vi "Push_OnlyPump.vi"(6 "Control":enum16{"First", "Second"}(ring), 10 "Port 1 in":T1={"Давление заданное"=0.3, "Давление MAX заданное"=100.0, "Давление в насосе"=0.0, "Давление в системе"=99.99, "Расход заданый"=0.0, "Расход текущий"=0.0, "Объём заданный"=0.0, "Объём текущий"=0.0, "Позиция насоса %"=0.0, "Ток двигателя"=0.0, "controlMsg"="", "Клапан k_sys"=FALSE, "Клапан k_res"=FALSE, "Клапан k_air"=FALSE, "Вверх"=FALSE, "Домой"=FALSE, "Вниз"=FALSE, "Старт расход"=FALSE, "Старт давление"=FALSE, "Сброс объёма"=FALSE, "Сброс давления Рсис"=FALSE, "Сброс давления Рнас"=FALSE, "Bits"={"plc_control"=FALSE, "lag_control"=FALSE, "mstop_control"=FALSE, "st_home"=FALSE, "error"=FALSE, "mstart"=FALSE, "pair"=FALSE, "startQ"=FALSE, "startP"=FALSE, "volume_Stop"=FALSE}} {"Ток двигателя" format="%#_5f"; "Расход текущий" format="%#_5f"; "Давление в системе" format="%.3f"; "Объём текущий" min=0.0 max=9999.0 step=0.0001 format="%#_5f"; "Объём заданный" min=0.0 max=9999.0 step=0.0001 format="%#_5f"; "Давление MAX заданное" min=0.0 max=100.0 step=0.01 format="%#_5f"; "Давление заданное" min=0.3 max=100.0 step=0.01 format="%#_5f"; "Расход заданый" min=0.0 max=40.0 step=0.0001 format="%#_5f"; "Давление в насосе" format="%.3f"; "Позиция насоса %" scale=0.0..100.0 scale format="%.2f"}, 11 "Управление ПЛК":T2) -> (3 "Port 1 out":T1={"Давление заданное"=0.3, "Давление MAX заданное"=100.0, "Давление в насосе"=0.0, "Давление в системе"=99.99, "Расход заданый"=0.0, "Расход текущий"=0.0, "Объём заданный"=0.0, "Объём текущий"=0.0, "Позиция насоса %"=0.0, "Ток двигателя"=0.0, "controlMsg"="", "Клапан k_sys"=FALSE, "Клапан k_res"=FALSE, "Клапан k_air"=FALSE, "Вверх"=FALSE, "Домой"=FALSE, "Вниз"=FALSE, "Старт расход"=FALSE, "Старт давление"=FALSE, "Сброс объёма"=FALSE, "Сброс давления Рсис"=FALSE, "Сброс давления Рнас"=FALSE, "Bits"={"plc_control"=FALSE, "lag_control"=FALSE, "mstop_control"=FALSE, "st_home"=FALSE, "error"=FALSE, "mstart"=FALSE, "pair"=FALSE, "startQ"=FALSE, "startP"=FALSE, "volume_Stop"=FALSE}} {"Ток двигателя" format="%#_5f"; "Расход текущий" format="%#_5f"; "Давление в системе" format="%.3f"; "Объём текущий" min=0.0 max=9999.0 step=0.0001 format="%#_5f"; "Объём заданный" min=0.0 max=9999.0 step=0.0001 format="%#_5f"; "Давление MAX заданное" min=0.0 max=100.0 step=0.01 format="%#_5f"; "Давление заданное" min=0.3 max=100.0 step=0.01 format="%#_5f"; "Расход заданый" min=0.0 max=40.0 step=0.0001 format="%#_5f"; "Давление в насосе" format="%.3f"; "Позиция насоса %" scale=0.0..100.0 scale format="%.2f"})   [LabVIEW 2018, in "pump_Lib.lvlib"]
uses:
  pump_Lib.lvlib
  TypeDef/control_Type.ctl
  TypeDef/pump_Type.ctl
  TypeDef/pair_Type.ctl
  Graph_data_collector/Stop event Type.ctl
  Scheduler/Stop Argument--cluster.ctl
  TypeDef/parametrs_Type.ctl
  Scheduler/Scheduler Lib.lvlib
panel:
  out "timed out?":bool
  # "%"
  # "%"
  # "%"
  # "%"
  # "%"
  # "%"
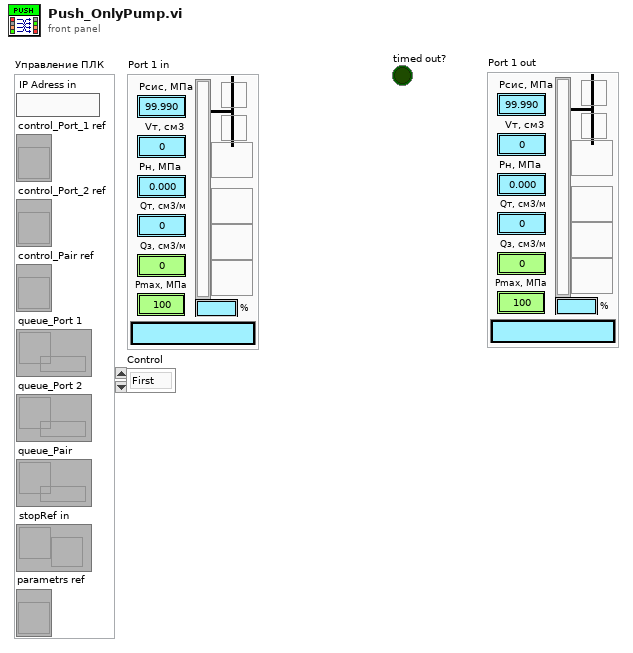
[diagram p1: front panel]
types:
  T1 = typedef "pump_Lib.lvlib/pump_Type.ctl" = cluster{"Давление заданное":dbl, "Давление MAX заданное":dbl, "Давление в насосе":dbl, "Давление в системе":dbl, "Расход заданый":dbl, "Расход текущий":dbl, "Объём заданный":dbl, "Объём текущий":dbl, "Позиция насоса %":dbl, "Ток двигателя":dbl, "controlMsg":string, "Клапан k_sys":bool, "Клапан k_res":bool, "Клапан k_air":bool, "Вверх":bool, "Домой":bool, "Вниз":bool, "Старт расход":bool, "Старт давление":bool, "Сброс объёма":bool, "Сброс давления Рсис":bool, "Сброс давления Рнас":bool, "Bits":cluster{"plc_control":bool, "lag_control":bool, "mstop_control":bool, "st_home":bool, "error":bool, "mstart":bool, "pair":bool, "startQ":bool, "startP":bool, "volume_Stop":bool}}
  T2 = typedef "pump_Lib.lvlib/control_Type.ctl" = cluster{"IP Adress in":string, "control_Port_1 ref":refnum<vi>, "control_Port_2 ref":refnum<vi>, "control_Pair ref":refnum<vi>, "queue_Port 1":refnum<queue>, "queue_Port 2":refnum<queue>, "queue_Pair":refnum<queue>, "stopRef in":T3, "parametrs ref":refnum<vi>}
  T3 = typedef "Scheduler Lib.lvlib/Stop event Type.ctl" = refnum<user-event>
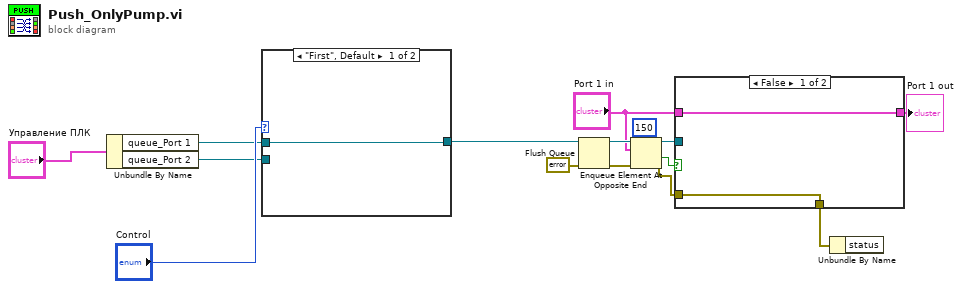
[diagram p0: block diagram]
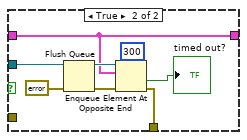
[diagram p3: hidden frame]
diagram:
  n1 = Unbundle By Name("Управление ПЛК") -> ("queue_Port 1"=w4:refnum<queue>, "queue_Port 2"=w6:refnum<queue>)
  n2 = case shown="\"First\", Default" "Control" {
    tunnel: w6 -> [_ w17]
    tunnel: [w16 w17] -> w5
    tunnel: w4 -> [w16 _]
    frame "First", Default {
    }
    frame "Second" {
    }
  }
  n3 = Flush Queue(queue=w5, error in (no error)=errorcluster {"status"=FALSE, "code"=0, "source"=""}) -> (queue out=w14:refnum<queue>, error out=w13:errorcluster)  [unwired: 1 out]
  n4 = Enqueue Element At Opposite End(queue=w14, element="Port 1 in", timeout in ms (-1)=150, error in (no error)=w13) -> (queue out=w11:refnum<queue>, timed out?=w3:bool, error out=w1:errorcluster)
  n5 = case shown="False" w3 {
    tunnel: w11 -> [_ w26]
    tunnel: "Port 1 in" -> [w19 w22]
    tunnel: [w19 w22] -> w8
    tunnel: [w18 w20] -> w2
    tunnel: w1 -> [w18 _]
    frame False {
    }
    frame True {
      n6 = Flush Queue(queue=w26, error in (no error)=errorcluster {"status"=FALSE, "code"=0, "source"=""}) -> (queue out=w23:refnum<queue>, error out=w27:errorcluster)  [unwired: 1 out]
      n7 = Enqueue Element At Opposite End(queue=w23, element=w22, timeout in ms (-1)=300, error in (no error)=w27) -> (timed out?=→"timed out?":bool, error out=w20:errorcluster)  [unwired: 1 out]
    }
  }
  "Port 1 out" <- w8
  n8 = Unbundle By Name(w2) -> ()  [unwired: 1 out]
